vi "task.vi"   [LabVIEW 2022 SP3, in "斯坦道多参数.lvlib"]
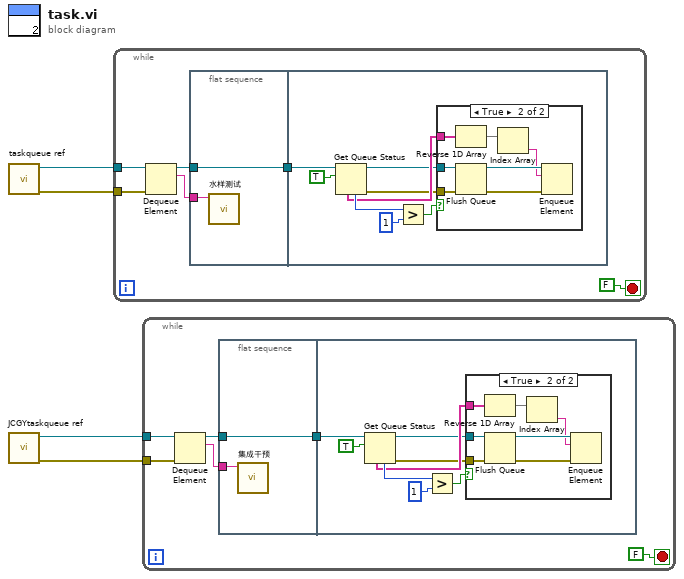
[diagram p0: block diagram]
diagram:
  n1 = call "taskqueue ref.vi"() -> ("错误输出"=w3:errorcluster, "队列输出"=w4:refnum<queue>)  [unwired: 10 in]
  n2 = call "JCGYtaskqueue ref.vi"() -> ("错误输出"=w1:errorcluster, "队列输出"=w2:refnum<queue>)  [unwired: 10 in]
  n3 = while {
    tunnel: w4 -> [w10]
    tunnel: w3 -> [w9]
    stop <- FALSE stop-if-true
    n4 = Dequeue Element(queue=w10, error in (no error)=w9) -> (queue out=w5:refnum<queue>, element=w7:string)  [unwired: 1 in, 2 out]
    n5 = flat-sequence {
      tunnel: w7 -> [w12]
      tunnel: [w11] -> w6
      tunnel: w5 -> [w11]
      tunnel: w6 -> [w20]
      frame #0 {
        n6 = call "水样测试.vi"("数据标记表"=w12) -> ()  [unwired: 11 in]
      }
      frame #1 {
        n7 = Get Queue Status(queue=w20, return elements? (F)=TRUE ("返回元素？(F)")) -> (queue out=w14:refnum<queue>, error out=w13:errorcluster, # elements in queue=w18:i32, elements=w15:string[])  [unwired: 1 in, 4 out]
        n8 = Greater?(x=w18, y=1) -> (0:w16:bool)
        n9 = case shown="True" w16 {
          tunnel: w15 -> [_ w27]
          tunnel: w14 -> [_ w25]
          tunnel: w13 -> [_ w24]
          frame False {
          }
          frame True {
            n10 = Reverse 1D Array(array=w27) -> (reversed array=w26:string[])
            n11 = Flush Queue(queue=w25, error in (no error)=w24) -> (queue out=w23:refnum<queue>, error out=w21:errorcluster)  [unwired: 1 out]
            n12 = Index Array(array=w26) -> (element=w22:string)  [unwired: 1 in]
            n13 = Enqueue Element(queue=w23, element=w22, error in (no error)=w21) -> ()  [unwired: 1 in, 3 out]
          }
        }
      }
    }
  }
  n14 = while {
    tunnel: w2 -> [w33]
    tunnel: w1 -> [w32]
    stop <- FALSE stop-if-true
    n15 = Dequeue Element(queue=w33, error in (no error)=w32) -> (queue out=w28:refnum<queue>, element=w30:string)  [unwired: 1 in, 2 out]
    n16 = flat-sequence {
      tunnel: w30 -> [w34]
      tunnel: [w35] -> w29
      tunnel: w28 -> [w35]
      tunnel: w29 -> [w43]
      frame #0 {
        n17 = call "集成干预.vi"("数据标记表"=w34) -> ()  [unwired: 11 in]
      }
      frame #1 {
        n18 = Get Queue Status(queue=w43, return elements? (F)=TRUE ("返回元素？(F)")) -> (queue out=w37:refnum<queue>, error out=w36:errorcluster, # elements in queue=w41:i32, elements=w38:string[])  [unwired: 1 in, 4 out]
        n19 = Greater?(x=w41, y=1) -> (0:w39:bool)
        n20 = case shown="True" w39 {
          tunnel: w38 -> [_ w50]
          tunnel: w37 -> [_ w48]
          tunnel: w36 -> [_ w47]
          frame False {
          }
          frame True {
            n21 = Reverse 1D Array(array=w50) -> (reversed array=w49:string[])
            n22 = Flush Queue(queue=w48, error in (no error)=w47) -> (queue out=w46:refnum<queue>, error out=w44:errorcluster)  [unwired: 1 out]
            n23 = Index Array(array=w49) -> (element=w45:string)  [unwired: 1 in]
            n24 = Enqueue Element(queue=w46, element=w45, error in (no error)=w44) -> ()  [unwired: 1 in, 3 out]
          }
        }
      }
    }
  }
